vi "Write Sampling Rate.vi"(8 "error in (no error)":errorcluster, 10 "Sampling Rate":T1=enum."30000Hz", 11 "LINX-ADS1X15 in":refnum<class "LINX-ADS1256.lvclass">) -> (0 "error out":errorcluster, 3 "LINX-ADS1X15 out":refnum<class "LINX-ADS1256.lvclass">)   [LabVIEW 2020, in "LINX-ADS1256.lvclass"]
uses:
  LINX-ADS1256.lvclass
  LINX-ADS1256.lvclass/LINX-ADS1256.ctl
  Sample Rate.ctl
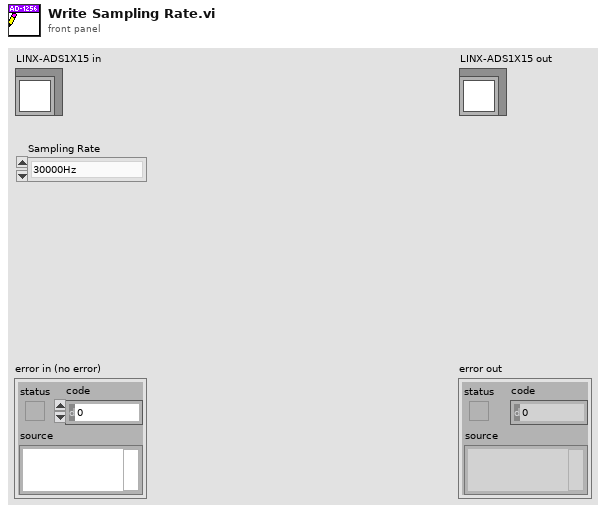
[diagram p1: front panel]
types:
  T1 = typedef "LINX-ADS1256.lvclass/Sample Rate.ctl" = enum16{"2.5Hz", "5Hz", "10Hz", "15Hz", "25Hz", "30Hz", "50Hz", "60Hz", "100Hz", "500Hz", "1000Hz", "2000Hz", "3750Hz", "7500Hz", "15000Hz", "30000Hz"}
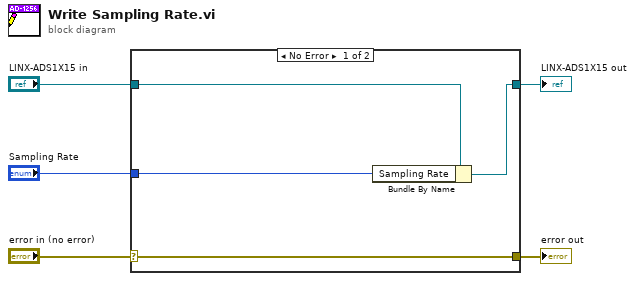
[diagram p0: block diagram]
diagram:
  n1 = case shown="No Error" "error in (no error)" {
    selector: "error in (no error)" -> [w9 w10]
    tunnel: [w9 w10] -> w4
    tunnel: [w7 w11] -> w2
    tunnel: "LINX-ADS1X15 in" -> [w8 w11]
    tunnel: "Sampling Rate" -> [w6 _]
    frame No Error {
      n2 = Bundle By Name(cluster=w8, "Sampling Rate"=w6) -> (w7:refnum<class "LINX-ADS1256.lvclass">)
    }
    frame Error {
    }
  }
  "error out" <- w4
  "LINX-ADS1X15 out" <- w2
